vi "solar_type Script to Message.vi"(6 "Array Delimiters (1D,2D)":string[](array[string]), 8 "error in (no error)":errorcluster, 11 "Script String":string) -> (0 "error out":errorcluster, 1 "Data":variant, 2 "Packet":string, 3 "Target":string, 4 "Remaining":string, 5 "Type":enum8{"CMD", "TLM"}(ring))   [LabVIEW 2018]
doc: "This converts a SOLAR script string to a variant message. Formatted as:\n<b>CMD|TLM.TARGET:PACKET{\nTYPE:VALUE,\nTYPE:'VALUE',\nTYPE|ENUM0|ENUM1|...:VALUE,\nTYPE_1D:'1,2,3',\nTYPE_2D:'1,2,3;4,5,6'}</b>\n\n<b>TYPE</b>= I8, I16, I32, I64, U8, U16, U32, U64, U8_ENUM, U16_ENUM, U32_ENUM, SGL, DBL, BOOL, STR, PATH, TIME\nTYPE_1D: 1D array (comma ',' delimited) Ex: DBL_1D:'1.23,4.567,8.92'\nTYPE_2D: 2D array (comma ',' & semicolon ';' delimited) Ex: I32_2D:'1,2,3;4,5,6'\nTYPE_ENUM: Enum with type items (pipe '|' delimited) Ex: U16_ENUM|Item 1|Item 2|Item 3:'Item 2'\n\nMyTarget:MyCMD{\nI32:-1234,\nSTR:'Hello World',\nU16_ENUM|Item1|Item2|Item3:'Item2',\nBOOL:true,\nTIME:'yyyy-mm-dd_hh:mm:ss.uuuuuu',\nPATH:'C:\\Data\\test.txt',\nU8_2D:'1,2,3;4,5,6'}"
panel:
  out "Debug Parameters":T1(array[cluster])
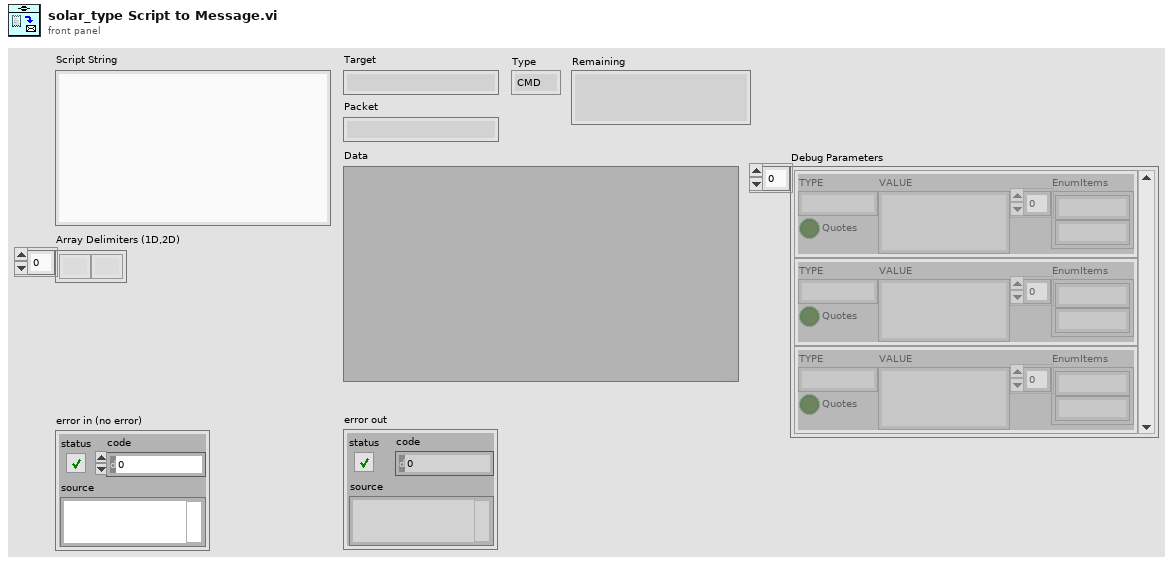
[diagram p1: front panel]
types:
  T1 = cluster{"TYPE":string, "VALUE":string, "Quotes":bool, "EnumItems":string[]}[]
  T2 = cluster{"TYPE":string, "VALUE":string, "Quotes":bool, "EnumItems":string[]}
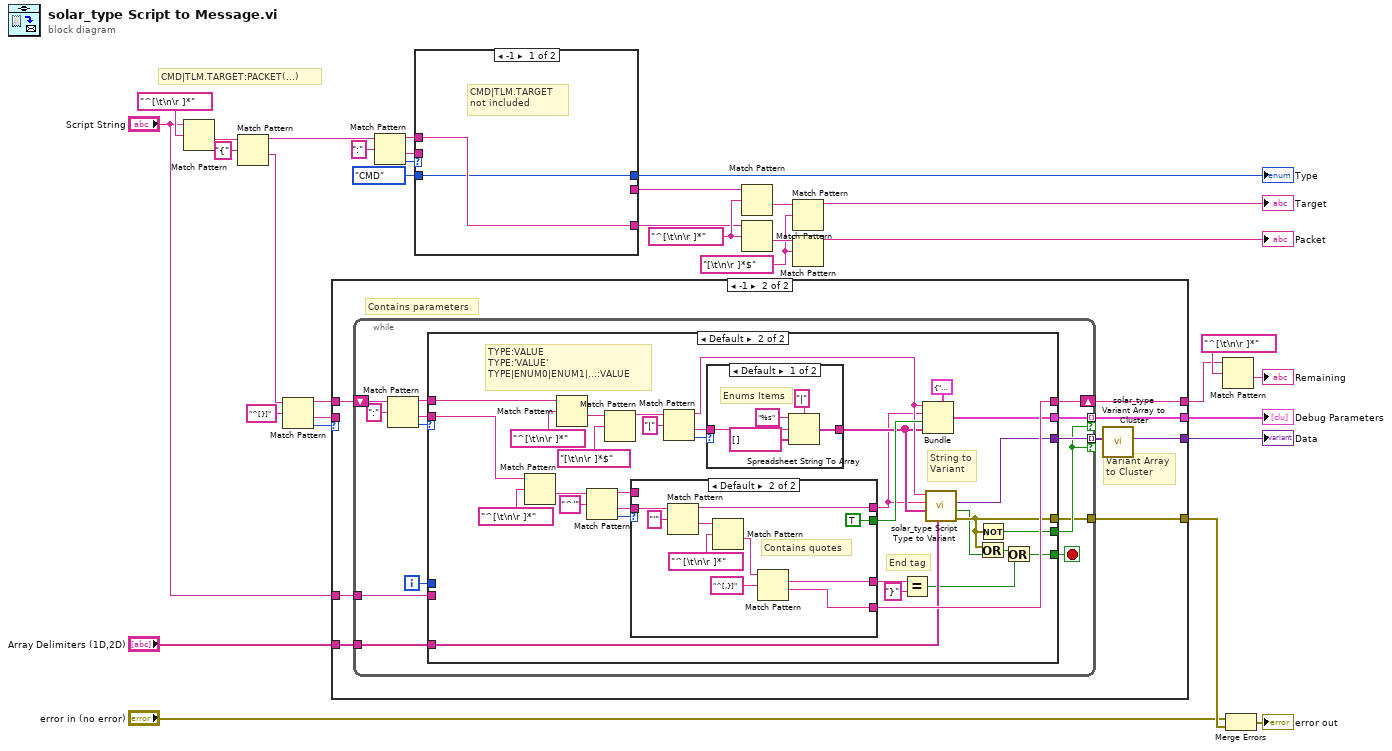
[diagram p0: block diagram]
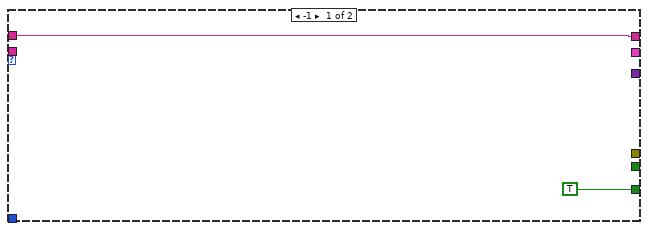
[diagram p3: hidden frame]
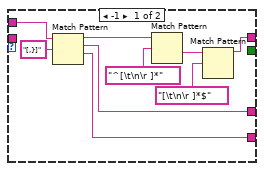
[diagram p5: hidden frame]
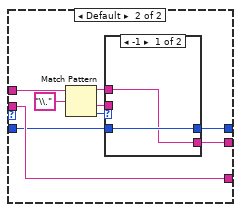
[diagram p6: hidden frame]
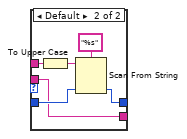
[diagram p7: hidden frame]
diagram:
  w15 = "[\t\n\r ]*$" ("regular expression")
  w16 = "^[\t\n\r ]*" ("regular expression")
  # "CMD|TLM.TARGET:PACKET(...)"
  n1 = Match Pattern(string="Script String", regular expression="^[\t\n\r ]*") -> (after substring=w30:string)  [unwired: 1 in, 3 out]
  n2 = Match Pattern(string=w30, regular expression="{") -> (before substring=w32:string, after substring=w4:string)  [unwired: 1 in, 2 out]
  n3 = Match Pattern(string=w4, regular expression="^[}]") -> (before substring=w3:string, after substring=w1:string, offset past match=w2:i32)  [unwired: 1 in, 1 out]
  n4 = case shown="-1" w2 {
    tunnel: w3 -> [_ w42]
    tunnel: [_ w41] -> w26
    tunnel: [_ w40] -> w25
    tunnel: "Script String" -> [_ w39]
    tunnel: [_ w37] -> w21
    tunnel: "Array Delimiters (1D,2D)" -> [_ w36]
    tunnel: [w34 w35] -> w7
    tunnel: w1 -> [w34 _]
    frame Default {
      # "Empty command\nPACKET{}"
    }
    frame -1 {
      # "Contains parameters"
      # "Variant Array\nto Cluster"
      n5 = while {
        shift-right: [w50] -> w35
        shift-left: w42 -> [w55]
        tunnel: [w51] -> w41 mode=indexing if=w47
        tunnel: [w48] -> w38 mode=indexing if=w47
        tunnel: [w46] -> w40
        tunnel: w39 -> [w44]
        tunnel: w36 -> [w43]
        i -> [w45]
        stop <- w49 stop-if-true
        n6 = Match Pattern(string=w55, regular expression=":") -> (before substring=w54:string, after substring=w52:string, offset past match=w53:i32)  [unwired: 1 in, 1 out]
        n7 = case shown="Default" w53 {
          tunnel: w54 -> [w57 w90]
          tunnel: w52 -> [_ w89]
          tunnel: [_ w87] -> w51
          tunnel: [w57 w88] -> w50
          tunnel: [_ w85] -> w47
          tunnel: [TRUE w60] -> w49
          tunnel: [_ w86] -> w48
          tunnel: [_ w83] -> w46
          tunnel: w45 -> [_ _]
          tunnel: w44 -> [_ _]
          tunnel: w43 -> [_ w63]
          frame -1 {
          }
          frame Default {
            # "End tag"
            # "String to\nVariant"
            # "TYPE:VALUE\nTYPE:'VALUE'\nTYPE|ENUM0|ENUM1|...:VALUE"
            n8 = Match Pattern(string=w89, regular expression="^[\t\n\r ]*") -> (after substring=w77:string)  [unwired: 1 in, 3 out]
            n9 = Match Pattern(string=w90, regular expression="^[\t\n\r ]*") -> (after substring=w80:string)  [unwired: 1 in, 3 out]
            n10 = Match Pattern(string=w77, regular expression="^'") -> (before substring=w68:string, after substring=w75:string, offset past match=w76:i32)  [unwired: 1 in, 1 out]
            n11 = Match Pattern(string=w80, regular expression="[\t\n\r ]*$") -> (before substring=w74:string)  [unwired: 1 in, 3 out]
            n12 = case shown="Default" w76 {
              tunnel: w75 -> [_ w113]
              tunnel: [w98 w112] -> w65
              tunnel: [w103 w107] -> w88
              tunnel: [_ TRUE] -> w70
              tunnel: w68 -> [w97 _]
              tunnel: [w96 w105] -> w61
              frame -1 {
                n13 = Match Pattern(string=w97, regular expression="[,}]") -> (before substring=w99:string, match substring=w96:string, after substring=w103:string)  [unwired: 1 in, 1 out]
                n14 = Match Pattern(string=w99, regular expression="^[\t\n\r ]*") -> (after substring=w102:string)  [unwired: 1 in, 3 out]
                n15 = Match Pattern(string=w102, regular expression="[\t\n\r ]*$") -> (before substring=w98:string)  [unwired: 1 in, 3 out]
              }
              frame Default {
                # "Contains quotes"
                n16 = Match Pattern(string=w113, regular expression="'") -> (before substring=w112:string, after substring=w110:string)  [unwired: 1 in, 2 out]
                n17 = Match Pattern(string=w110, regular expression="^[\t\n\r ]*") -> (after substring=w108:string)  [unwired: 1 in, 3 out]
                n18 = Match Pattern(string=w108, regular expression="^[,}]") -> (match substring=w105:string, after substring=w107:string)  [unwired: 1 in, 2 out]
              }
            }
            n19 = Match Pattern(string=w74, regular expression="|") -> (before substring=w67:string, after substring=w71:string, offset past match=w72:i32)  [unwired: 1 in, 1 out]
            n20 = case shown="Default" w72 {
              tunnel: w71 -> [w91 _]
              tunnel: [w92 _] -> w66
              frame Default {
                # "Enums Items"
                n21 = Spreadsheet String To Array(delimiter (Tab)="|", format string="%s", spreadsheet string=w91, array type (2D Dbl)=string[] []) -> (array=w92:string[])
              }
              frame -1 {
              }
            }
            n22 = Equal?(x=w61, y="}") -> (x = y?=w59:bool)
            n23 = Bundle(cluster=T2 {"TYPE"="", "VALUE"="", "Quotes"=FALSE, "EnumItems"=[]} ("PARAMETER"), "TYPE"=w67, "VALUE"=w65, "Quotes"=w70, "EnumItems"=w66) -> (w87:T2)
            n24 = call "solar_type Script Type to Variant.vi"("Array Delimiters (1D,2D)"=w63, "EnumItems"=w66, "Value String"=w65, "Type String"=w67) -> ("error out"=w83:errorcluster, "Invalid?"=w64:bool, "Value Variant"=w86:variant)  [unwired: 4 in, 1 out]
            n25 = Not(x=w83) -> (.not. x?=w85:bool)
            n26 = Or(x=w83, y=w64) -> (x .or. y?=w84:bool)
            n27 = Or(x=w84, y=w59) -> (x .or. y?=w60:bool)
          }
        }
      }
      n28 = call "solar_type Variant Array to Cluster.vi"("Variant Elements"=w38) -> ("Cluster Variant"=w37:variant)  [unwired: 10 in]
    }
  }
  "Debug Parameters" <- w26
  "Data" <- w21
  n29 = Match Pattern(string=w32, regular expression=":") -> (before substring=w14:string, after substring=w11:string, offset past match=w10:i32)  [unwired: 1 in, 1 out]
  n30 = case shown="-1" w10 {
    tunnel: [w115 w125] -> w28
    tunnel: w14 -> [w116 w123]
    tunnel: [_ w119] -> w13
    tunnel: [w116 w118] -> w12
    tunnel: w11 -> [_ w118]
    tunnel: enum8{"CMD", "TLM"}."CMD" ("Type") -> [w115 w117]
    frame -1 {
      # "CMD|TLM.TARGET\nnot included"
    }
    frame Default {
      n31 = Match Pattern(string=w123, regular expression="\\.") -> (before substring=w122:string, after substring=w120:string, offset past match=w121:i32)  [unwired: 1 in, 1 out]
      n32 = case shown="-1" w121 {
        tunnel: w117 -> [w127 w132]
        tunnel: [w127 w131] -> w125
        tunnel: w122 -> [w126 w129]
        tunnel: w120 -> [_ w128]
        tunnel: [w126 w128] -> w119
        frame -1 {
        }
        frame Default {
          n33 = To Upper Case(1:w129) -> (0:w133:string)
          n34 = Scan From String(format string="%s", input string=w133, default 1=w132) -> (output 1=w131:enum8{"CMD", "TLM"})  [unwired: 2 in, 3 out]
        }
      }
    }
  }
  "Type" <- w28
  n35 = Match Pattern(string=w13, regular expression=w16) -> (after substring=w17:string)  [unwired: 1 in, 3 out]
  n36 = Match Pattern(string=w12, regular expression=w16) -> (after substring=w18:string)  [unwired: 1 in, 3 out]
  n37 = Match Pattern(string=w17, regular expression=w15) -> (before substring=→"Target":string)  [unwired: 1 in, 3 out]
  n38 = Match Pattern(string=w18, regular expression=w15) -> (before substring=→"Packet":string)  [unwired: 1 in, 3 out]
  n39 = Match Pattern(string=w7, regular expression="^[\t\n\r ]*") -> (after substring=→"Remaining":string)  [unwired: 1 in, 3 out]
  n40 = Merge Errors("error in (no error)", w25) -> (→"error out":errorcluster)
